vi "Update Segment.vi"(0 "TreeNode in":refnum<class "TreeNode.lvclass">, 1 "Start":refnum<class "Data.lvclass">, 2 "End":refnum<class "Data.lvclass">, 3 "Dimension":refnum<class "Data.lvclass">, 5 "error in (no error)":errorcluster) -> (14 "TreeNode out":refnum<class "TreeNode.lvclass">, 19 "error out":errorcluster)   [LabVIEW 2015, in "MDSplus.lvlib" / "TreeNode.lvclass"]
uses:
  <userlib>/MDSplus/Classes/Data_Class/TreeNode_Class/TreeNode.lvclass
  <userlib>/MDSplus/Classes/Data_Class/Data.lvclass
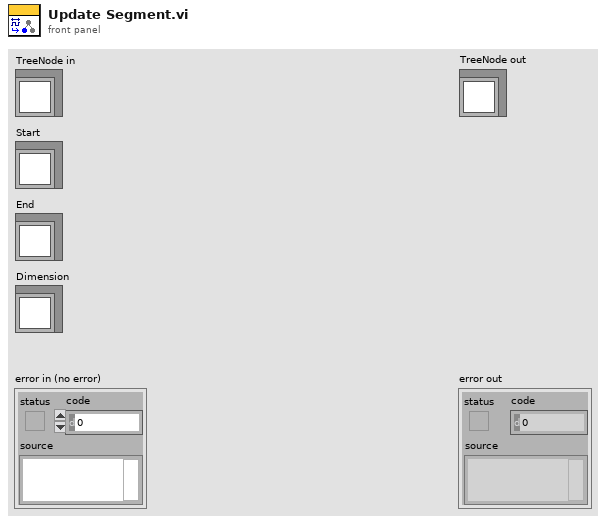
[diagram p1: front panel]
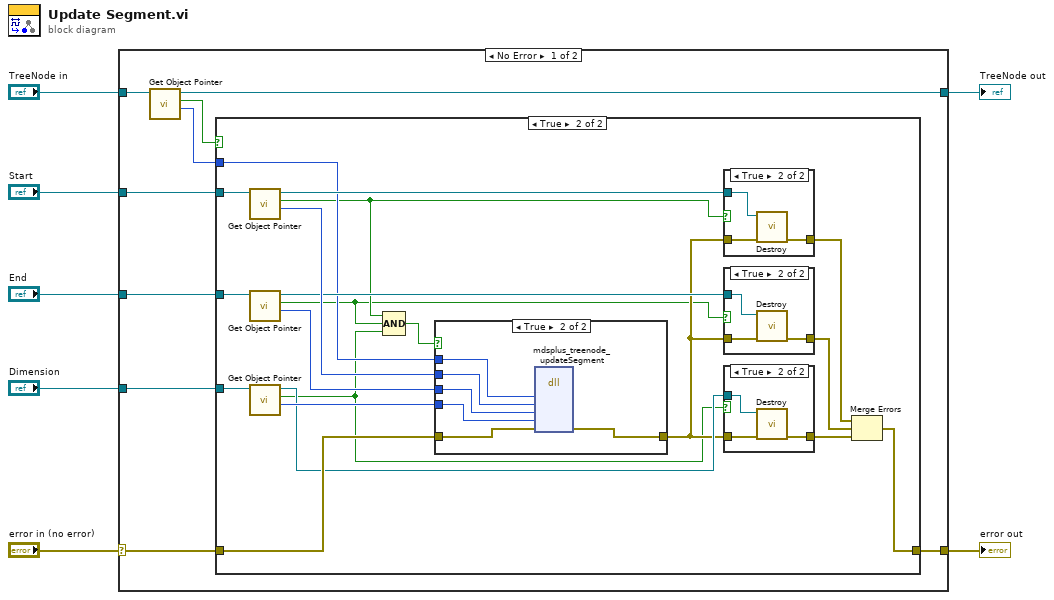
[diagram p0: block diagram]
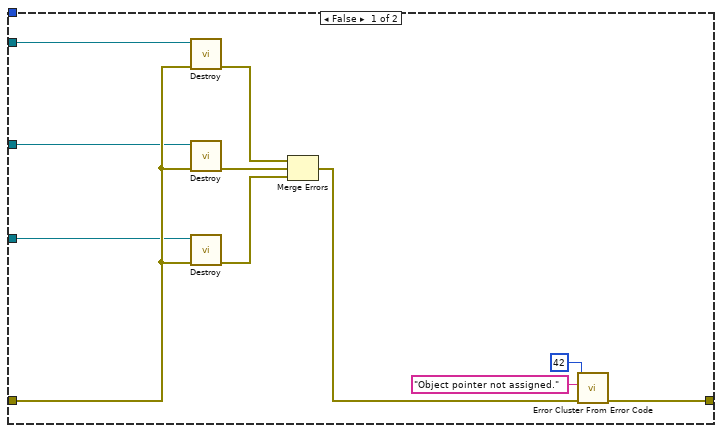
[diagram p2: hidden frame]
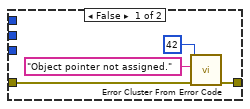
[diagram p6: hidden frame]
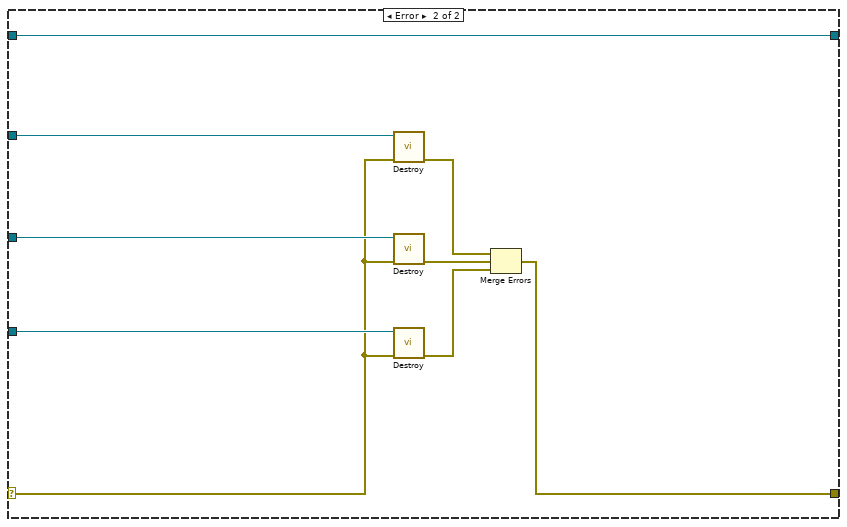
[diagram p7: hidden frame]
diagram:
  n1 = case shown="No Error" "error in (no error)" {
    selector: "error in (no error)" -> [w13 w70]
    tunnel: [w12 w71] -> w6
    tunnel: [w10 w78] -> w5
    tunnel: "TreeNode in" -> [w11 w78]
    tunnel: "Start" -> [w16 w77]
    tunnel: "End" -> [w15 w76]
    tunnel: "Dimension" -> [w14 w75]
    frame No Error {
      n2 = call-dynamic "Get Object Pointer.vi"("Data in"=w11) -> ("Object Pointer"=w8:i64, "Assigned object pointer?"=w9:bool, "Data out"=w10:refnum<class "TreeNode.lvclass">)  [unwired: 8 in]
      n3 = case shown="True" w9 {
        tunnel: w16 -> [w24 w47]
        tunnel: w15 -> [w22 w46]
        tunnel: w14 -> [w21 w45]
        tunnel: w13 -> [w23 w41]
        tunnel: [w17 w34] -> w12
        tunnel: w8 -> [_ w31]
        frame False {
          n4 = call-dynamic "Destroy.vi"("error in (no error)"=w23, "Data in"=w24) -> ("error out"=w25:errorcluster)  [unwired: 9 in]
          n5 = call-dynamic "Destroy.vi"("error in (no error)"=w23, "Data in"=w22) -> ("error out"=w27:errorcluster)  [unwired: 9 in]
          n6 = call-dynamic "Destroy.vi"("error in (no error)"=w23, "Data in"=w21) -> ("error out"=w26:errorcluster)  [unwired: 9 in]
          n7 = Merge Errors(w25, w27, w26) -> (w18:errorcluster)
          n8 = call <vilib>:"Error Cluster From Error Code.vi"("error in (no error)"=w18, "error message (\"\")"="Object pointer not assigned." ("error message (\"\")"), "error code (0)"=42) -> ("error out"=w17:errorcluster)  [unwired: 6 in]
        }
        frame True {
          n9 = call-dynamic "Get Object Pointer.vi"("Data in"=w47) -> ("Object Pointer"=w42:i64, "Assigned object pointer?"=w30:bool, "Data out"=w40:refnum<class "Data.lvclass">)  [unwired: 8 in]
          n10 = call-dynamic "Get Object Pointer.vi"("Data in"=w46) -> ("Object Pointer"=w43:i64, "Assigned object pointer?"=w29:bool, "Data out"=w39:refnum<class "Data.lvclass">)  [unwired: 8 in]
          n11 = call-dynamic "Get Object Pointer.vi"("Data in"=w45) -> ("Object Pointer"=w44:i64, "Assigned object pointer?"=w28:bool, "Data out"=w38:refnum<class "Data.lvclass">)  [unwired: 8 in]
          n12 = Compound Arithmetic op=AND(w30, w29, w28) -> (w33:bool)
          n13 = case shown="True" w33 {
            tunnel: w44 -> [_ w69]
            tunnel: w43 -> [_ w68]
            tunnel: w42 -> [_ w67]
            tunnel: w41 -> [w61 w66]
            tunnel: [w60 w65] -> w32
            tunnel: w31 -> [_ w64]
            frame False {
              n14 = call <vilib>:"Error Cluster From Error Code.vi"("error in (no error)"=w61, "error message (\"\")"="Object pointer not assigned." ("error message (\"\")"), "error code (0)"=42) -> ("error out"=w60:errorcluster)  [unwired: 6 in]
            }
            frame True {
              n15 = dll-call lib="MDSobjectsLVShr" fn="mdsplus_treenode_updateSegment"("lvTreeNodePtr"=w64, "lvStartDataPtrIn"=w67, "lvEndDataPtrIn"=w68, "lvTimeDataPtrIn"=w69, "error"=w66) -> ("error"=w65:errorcluster)  [unwired: 8 in, 2 out]
            }
          }
          n16 = case shown="True" w30 {
            tunnel: w32 -> [w52 w55]
            tunnel: w40 -> [_ w54]
            tunnel: [w52 w53] -> w35
            frame False {
            }
            frame True {
              n17 = call-dynamic "Destroy.vi"("error in (no error)"=w55, "Data in"=w54) -> ("error out"=w53:errorcluster)  [unwired: 9 in]
            }
          }
          n18 = case shown="True" w29 {
            tunnel: w32 -> [w56 w59]
            tunnel: w39 -> [_ w58]
            tunnel: [w56 w57] -> w36
            frame False {
            }
            frame True {
              n19 = call-dynamic "Destroy.vi"("error in (no error)"=w59, "Data in"=w58) -> ("error out"=w57:errorcluster)  [unwired: 9 in]
            }
          }
          n20 = case shown="True" w28 {
            tunnel: w32 -> [w48 w51]
            tunnel: w38 -> [_ w50]
            tunnel: [w48 w49] -> w37
            frame False {
            }
            frame True {
              n21 = call-dynamic "Destroy.vi"("error in (no error)"=w51, "Data in"=w50) -> ("error out"=w49:errorcluster)  [unwired: 9 in]
            }
          }
          n22 = Merge Errors(w35, w36, w37) -> (w34:errorcluster)
        }
      }
    }
    frame Error {
      n23 = call-dynamic "Destroy.vi"("error in (no error)"=w70, "Data in"=w77) -> ("error out"=w72:errorcluster)  [unwired: 9 in]
      n24 = call-dynamic "Destroy.vi"("error in (no error)"=w70, "Data in"=w76) -> ("error out"=w74:errorcluster)  [unwired: 9 in]
      n25 = call-dynamic "Destroy.vi"("error in (no error)"=w70, "Data in"=w75) -> ("error out"=w73:errorcluster)  [unwired: 9 in]
      n26 = Merge Errors(w72, w74, w73) -> (w71:errorcluster)
    }
  }
  "error out" <- w6
  "TreeNode out" <- w5
